vi "Reconfigurable ConfigManager.vi"() -> ()   [LabVIEW 2014]
uses:
  ModuleA class/Configuration - cluster.ctl
  <vilib>/LabVIEW Open Source Project/Configuration Manager/Encoding.Base64/Encoding.Base64.lvclass
  <vilib>/LabVIEW Open Source Project/Configuration Manager/Manager.Text/ConfigManager.Text.lvclass
  <vilib>/LabVIEW Open Source Project/Unicity/Delimiter/Delimiters List.ctl
  <vilib>/LabVIEW Open Source Project/Configuration Manager/Manager/ConfigManager.lvclass/ConfigManager.ctl
  <vilib>/LabVIEW Open Source Project/Configuration Manager/Manager.Text/ConfigManager.Text.lvclass/ConfigManager.Text.ctl
  <vilib>/JKI/JKI SMO/SMO/SMO.lvclass
  ModuleA class/ModuleA.lvclass
  <vilib>/LabVIEW Open Source Project/Configuration Manager/Manager/ConfigManager.lvclass
  <vilib>/LabVIEW Open Source Project/Unicity/Delimiter/Delimiter.lvclass
panel:
  out "Module C":T1
  out "Module B":T1
  out "Module A":T1
  out "error out":errorcluster
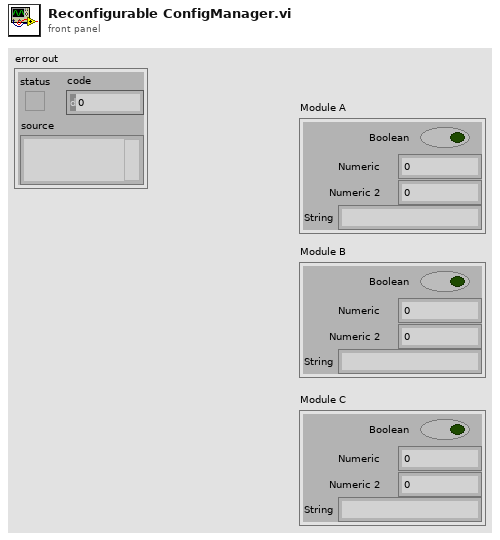
[diagram p1: front panel]
types:
  T1 = typedef "ModuleA.lvclass/Configuration - cluster.ctl" = cluster{"Boolean":bool, "Numeric":dbl, "Numeric 2":dbl, "String":string}
  T2 = typedef "Delimiter.lvclass/Delimiters List.ctl" = enum16{"Default", "dot (.)", "colon (:)", "double-colon (::)", "semi-colon (;)", "underscore (_)", "double underscore (__)", "dash (-)", "double dash (--)", "backslash (\\)", "vertical bar (|)", "forward slash (/)", "chevron (>)", "double-chevron (>>)", "arrow (->)", "comma (,)", "arobas (@)", "ampersand (&)", "other"}
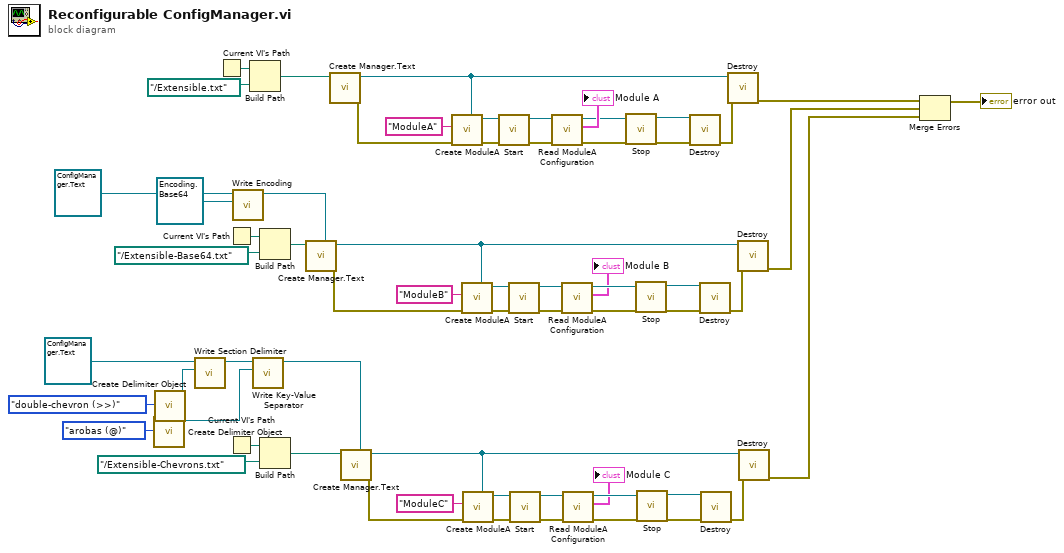
[diagram p0: block diagram]
diagram:
  n1 = call <vilib>:"Create Delimiter Object.vi"("Delimiter"=Delimiters_List."arobas (@)") -> ("Delimiter"=w4:refnum<class "Delimiter.lvclass">)  [unwired: 10 in]
  n2 = call <vilib>:"Create Delimiter Object.vi"("Delimiter"=Delimiters_List."double-chevron (>>)") -> ("Delimiter"=w8:refnum<class "Delimiter.lvclass">)  [unwired: 10 in]
  n3 = call <vilib>:"Write Section Delimiter.vi"("Section Delimiter"=w8, "ConfigManager.Text in"=refnum<class "ConfigManager.Text.lvclass"> refnum ("ConfigManager.Text")) -> ("ConfigManager.Text out"=w6:refnum<class "ConfigManager.Text.lvclass">)  [unwired: 9 in]
  n4 = Current VI's Path() -> (path=w60:path)
  n5 = Current VI's Path() -> (path=w32:path)
  n6 = Current VI's Path() -> (path=w11:path)
  n7 = call <vilib>:"Write Encoding.vi"("Encoding"=refnum<class "Encoding.Base64.lvclass"> refnum ("CfgEncoding in"), "ConfigManager in"=refnum<class "ConfigManager.Text.lvclass"> refnum ("ConfigManager.Text")) -> ("ConfigManager out"=w26:refnum<class "ConfigManager.Text.lvclass">)  [unwired: 9 in]
  n8 = Build Path(base path=w60, name or relative path=path "../Extensible.txt") -> (appended path=w61:path)
  n9 = call <vilib>:"Write Key-Value Separator.vi"("Key Value Delimiter"=w4, "ConfigManager.Text in"=w6) -> ("ConfigManager.Text out"=w3:refnum<class "ConfigManager.Text.lvclass">)  [unwired: 9 in]
  n10 = Build Path(base path=w32, name or relative path=path "../Extensible-Base64.txt") -> (appended path=w31:path)
  n11 = Build Path(base path=w11, name or relative path=path "../Extensible-Chevrons.txt") -> (appended path=w10:path)
  n12 = call <vilib>:"Create Manager.Text.vi"("ConfigManager.Text"=w26, "filepath"=w31) -> ("error out"=w34:errorcluster, "ConfigManager.Text out"=w25:refnum<class "ConfigManager.Text.lvclass">)  [unwired: 7 in, 1 out]
  n13 = call <vilib>:"Create Manager.Text.vi"("filepath"=w61) -> ("error out"=w58:errorcluster, "ConfigManager.Text out"=w57:refnum<class "ConfigManager.Text.lvclass">)  [unwired: 8 in, 1 out]
  n14 = call <vilib>:"Create Manager.Text.vi"("ConfigManager.Text"=w3, "filepath"=w10) -> ("error out"=w13:errorcluster, "ConfigManager.Text out"=w14:refnum<class "ConfigManager.Text.lvclass">)  [unwired: 7 in, 1 out]
  n15 = call "Create ModuleA.vi"("ConfigManager"=w57, "error in (no error)"=w58, "Subsystem Name (optional)"="ModuleA") -> ("error out"=w53:errorcluster, "ModuleA out"=w54:refnum<class "ModuleA.lvclass">)  [unwired: 6 in, 1 out]
  n16 = call "Create ModuleA.vi"("ConfigManager"=w25, "error in (no error)"=w34, "Subsystem Name (optional)"="ModuleB") -> ("error out"=w38:errorcluster, "ModuleA out"=w37:refnum<class "ModuleA.lvclass">)  [unwired: 6 in, 1 out]
  n17 = call "Create ModuleA.vi"("ConfigManager"=w14, "error in (no error)"=w13, "Subsystem Name (optional)"="ModuleC") -> ("error out"=w18:errorcluster, "ModuleA out"=w17:refnum<class "ModuleA.lvclass">)  [unwired: 6 in, 1 out]
  n18 = call <vilib>:"Start.vi"("error in (no error)"=w53, "SMO"=w54) -> ("error out"=w51:errorcluster, "SMO out"=w52:refnum<class "ModuleA.lvclass">)  [unwired: 8 in]
  n19 = call <vilib>:"Start.vi"("error in (no error)"=w38, "SMO"=w37) -> ("error out"=w40:errorcluster, "SMO out"=w39:refnum<class "ModuleA.lvclass">)  [unwired: 8 in]
  n20 = call <vilib>:"Start.vi"("error in (no error)"=w18, "SMO"=w17) -> ("error out"=w20:errorcluster, "SMO out"=w19:refnum<class "ModuleA.lvclass">)  [unwired: 8 in]
  n21 = call "Read ModuleA Configuration.vi"("error in (no error)"=w51, "ModuleA in"=w52) -> ("error out"=w49:errorcluster, "Configuration"=→"Module A":T1, "ModuleA out"=w50:refnum<class "ModuleA.lvclass">)  [unwired: 7 in]
  n22 = call "Read ModuleA Configuration.vi"("error in (no error)"=w40, "ModuleA in"=w39) -> ("error out"=w42:errorcluster, "Configuration"=→"Module B":T1, "ModuleA out"=w41:refnum<class "ModuleA.lvclass">)  [unwired: 7 in]
  n23 = call "Read ModuleA Configuration.vi"("error in (no error)"=w20, "ModuleA in"=w19) -> ("error out"=w22:errorcluster, "Configuration"=→"Module C":T1, "ModuleA out"=w21:refnum<class "ModuleA.lvclass">)  [unwired: 7 in]
  n24 = call <vilib>:"Stop.vi"("error in (no error)"=w49, "SMO"=w50) -> ("error out"=w47:errorcluster, "SMO out"=w48:refnum<class "ModuleA.lvclass">)  [unwired: 8 in]
  n25 = call <vilib>:"Stop.vi"("error in (no error)"=w42, "SMO"=w41) -> ("error out"=w44:errorcluster, "SMO out"=w43:refnum<class "ModuleA.lvclass">)  [unwired: 8 in]
  n26 = call <vilib>:"Stop.vi"("error in (no error)"=w22, "SMO"=w21) -> ("error out"=w24:errorcluster, "SMO out"=w23:refnum<class "ModuleA.lvclass">)  [unwired: 8 in]
  n27 = call <vilib>:"Destroy.vi"("error in (no error)"=w47, "SMO"=w48) -> ("error out"=w56:errorcluster)  [unwired: 9 in]
  n28 = call <vilib>:"Destroy.vi"("error in (no error)"=w44, "SMO"=w43) -> ("error out"=w35:errorcluster)  [unwired: 9 in]
  n29 = call <vilib>:"Destroy.vi"("error in (no error)"=w24, "SMO"=w23) -> ("error out"=w15:errorcluster)  [unwired: 9 in]
  n30 = call-dynamic <vilib>:"Destroy.vi"("error in (no error)"=w56, "ConfigManager.Text in"=w57) -> ("error out"=w46:errorcluster)  [unwired: 8 in, 1 out]
  n31 = call-dynamic <vilib>:"Destroy.vi"("error in (no error)"=w35, "ConfigManager.Text in"=w25) -> ("error out"=w29:errorcluster)  [unwired: 8 in, 1 out]
  n32 = call-dynamic <vilib>:"Destroy.vi"("error in (no error)"=w15, "ConfigManager.Text in"=w14) -> ("error out"=w2:errorcluster)  [unwired: 8 in, 1 out]
  n33 = Merge Errors(w46, w29, w2) -> (→"error out":errorcluster)
